vi "Configure Sample Rate [ARB] Core.vi"(8 "error in (no error)":errorcluster, 9 "sample rate (1000 Samp/s)":dbl[unit]=1000.0 format="%^.2e", 11 "IVI_Fgen in":refnum<class "IVI_Fgen.lvclass">) -> (0 "error out":errorcluster, 3 "IVI_Fgen out":refnum<class "IVI_Fgen.lvclass">)   [LabVIEW 2015, in "IVI_Fgen.lvlib" / "IVI_Fgen.lvclass"]
doc: "This VI configures the rate at which the function generator produces the points that make up arbitrary waveforms. When you configure the function generator to produce an arbitrary sequence, this is the sample rate for all arbitrary waveforms in the sequence.\n \nNotes:\n\n(1) This VI is part of the IviFgenArbWfm [ARB] extension group."
uses:
  IVI_Fgen.lvclass
  IVI_Fgen.lvclass/IVI_Fgen.ctl
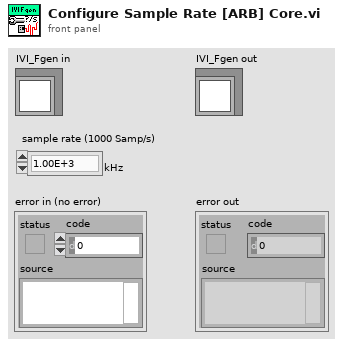
[diagram p1: front panel]
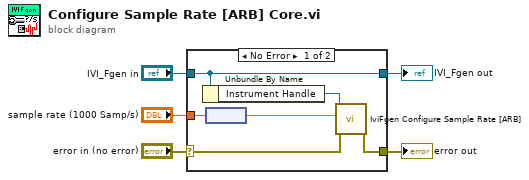
[diagram p0: block diagram]
diagram:
  n1 = case shown="No Error" "error in (no error)" {
    selector: "error in (no error)" -> [w9 w13]
    tunnel: [w8 w13] -> w4
    tunnel: [w11 w12] -> w2
    tunnel: "IVI_Fgen in" -> [w11 w12]
    tunnel: "sample rate (1000 Samp/s)" -> [w7 _]
    frame No Error {
      n2 = Unbundle By Name(w11) -> ("Instrument Handle"=w10:refnum<k15>)
      n3 = node(w7) -> (w6:dbl)
      n4 = call <vilib>:"IviFgen Configure Sample Rate [ARB].vi"("error in (no error)"=w9, "sample rate (1000 Samp/s)"=w6, "instrument handle"=w10) -> ("error out"=w8:errorcluster)  [unwired: 7 in, 1 out]
    }
    frame Error {
    }
  }
  "error out" <- w4
  "IVI_Fgen out" <- w2
